vi "Colour location on myRio.vi"() -> ()   [LabVIEW 2018]
panel:
  out "error out":errorcluster
  out "Frame Rate":dbl
  out "Number of Matches (SOAP)":i32
  out "Matches (SOAP)":T1(array[cluster]) {"Bounding Box"."y" format="%.2f"; "Bounding Box"."x" format="%.2f"; "Position"."y" format="%.2f"; "Position"."x" format="%.2f"; "Score" format="%.2f"; "Scale" format="%.2f"; "Angle" format="%.2f"}
  out "Number of Matches (BLACK)":i32
  out "Matches (BLACK)":T1(array[cluster]) {"Bounding Box"."y" format="%.2f"; "Bounding Box"."x" format="%.2f"; "Position"."y" format="%.2f"; "Position"."x" format="%.2f"; "Score" format="%.2f"; "Scale" format="%.2f"; "Angle" format="%.2f"}
  out "Number of Matches (RED)":i32
  out "Matches (RED)":T1(array[cluster]) {"Bounding Box"."y" format="%.2f"; "Bounding Box"."x" format="%.2f"; "Position"."y" format="%.2f"; "Position"."x" format="%.2f"; "Score" format="%.2f"; "Scale" format="%.2f"; "Angle" format="%.2f"}
  out "Number of Matches (GREY)":i32
  out "Matches (GREY)":T1(array[cluster]) {"Bounding Box"."y" format="%.2f"; "Bounding Box"."x" format="%.2f"; "Position"."y" format="%.2f"; "Position"."x" format="%.2f"; "Score" format="%.2f"; "Scale" format="%.2f"; "Angle" format="%.2f"}
  in  "Minimum Match Score (SOAP)":sgl=800.0
  in  "Minimum Match Score (BLACK)":sgl=800.0
  in  "Minimum Match Score (RED)":sgl=800.0
  in  "Minimum Match Score (GREY)":sgl=800.0
  in  "Stop (F)":bool
  out "Image Out":T2(plugin-control)
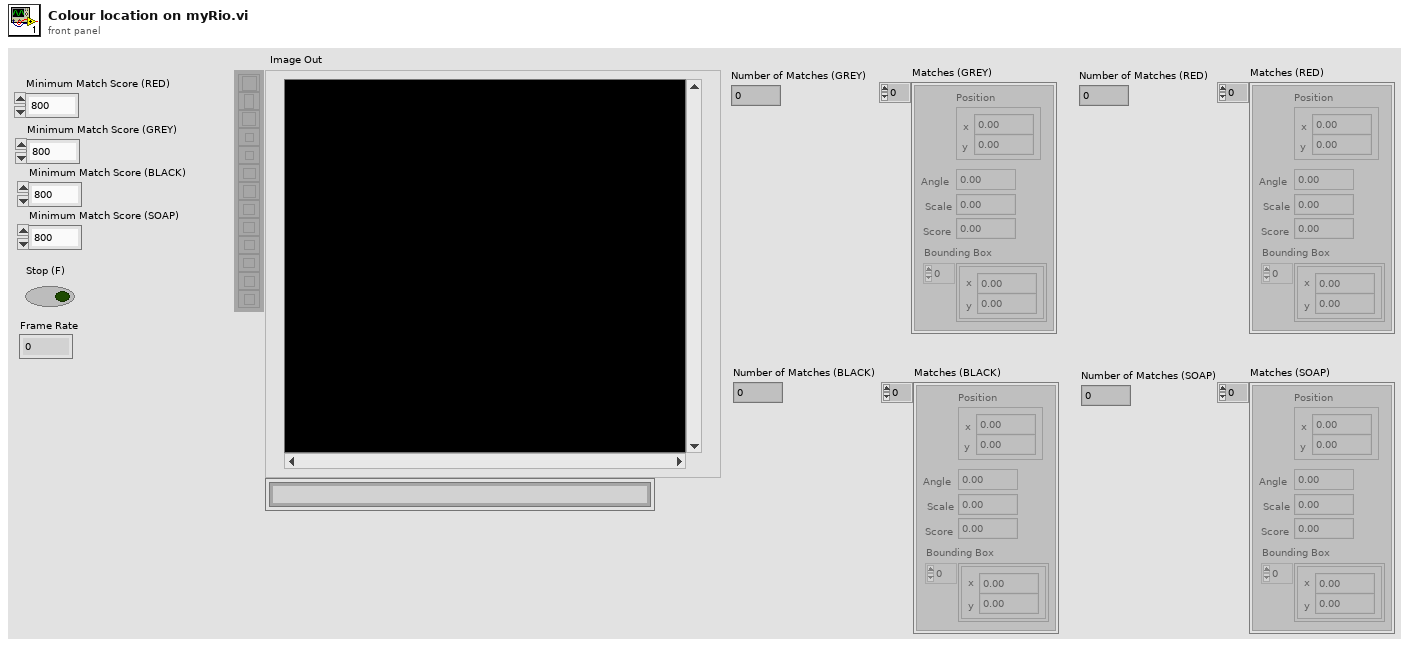
[diagram p1: front panel]
types:
  T1 = cluster{"Position":cluster{"x":sgl, "y":sgl}, "Angle":sgl, "Scale":sgl, "Score":sgl, "Bounding Box":cluster{"x":sgl, "y":sgl}[]}[]
  T2 = typedef "IMAQ Image.ctl" = refnum<image>
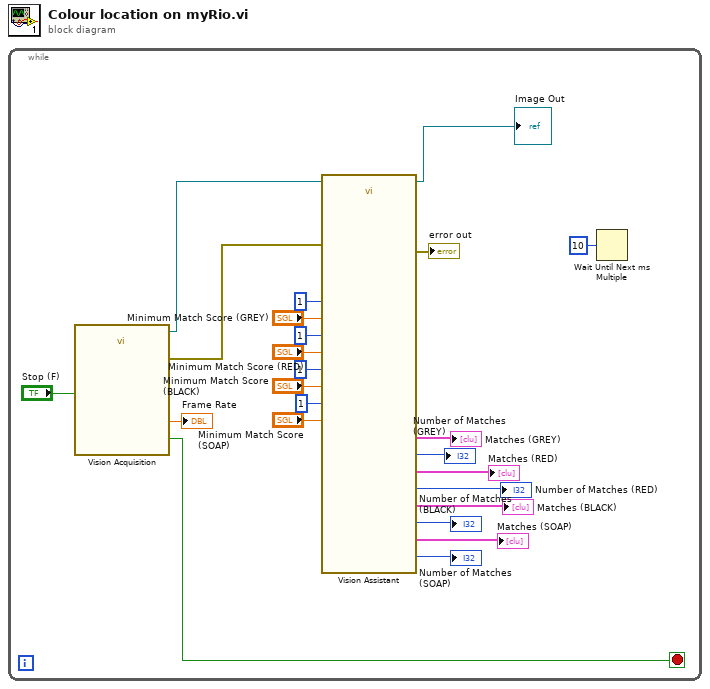
[diagram p0: block diagram]
diagram:
  n1 = while {
    stop <- w23 stop-if-true
    n2 = call "Vision Acquisition"("Stop (F)"="Stop (F)") -> ("Image Out"=w5:T2, "Frame Rate"=→"Frame Rate":dbl, "Stopped"=w23:bool, "error out"=w2:errorcluster)  [unwired: 23 in]
    n3 = call "Vision Assistant"("Image In"=w5, "Number of Matches Requested (GREY)"=1, "Minimum Match Score (GREY)"="Minimum Match Score (GREY)", "Number of Matches Requested (RED)"=1, "Minimum Match Score (RED)"="Minimum Match Score (RED)", "Number of Matches Requested (BLACK)"=1 ("Number of Matches Requested (RED)"), "error in"=w2, "Minimum Match Score (BLACK)"="Minimum Match Score (BLACK)", "Number of Matches Requested (SOAP)"=1 ("Number of Matches Requested (RED)"), "Minimum Match Score (SOAP)"="Minimum Match Score (SOAP)") -> ("Number of Matches (SOAP)"=→"Number of Matches (SOAP)":i32, "Matches (SOAP)"=→"Matches (SOAP)":T1, "Image Out"=→"Image Out":T2, "Matches (GREY)"=→"Matches (GREY)":T1, "Number of Matches (GREY)"=→"Number of Matches (GREY)":i32, "Matches (RED)"=→"Matches (RED)":T1, "Number of Matches (RED)"=→"Number of Matches (RED)":i32, "Matches (BLACK)"=→"Matches (BLACK)":T1, "Number of Matches (BLACK)"=→"Number of Matches (BLACK)":i32, "error out"=→"error out":errorcluster)  [unwired: 8 in]
    n4 = Wait Until Next ms Multiple(millisecond multiple=u32 10) -> ()  [unwired: 1 out]
  }
